vi "tare.vi"(0 "LC2 Tare\nAmount":dbl, 1 "Tare Pitot Tube\nNote: ONLY USE AT\nIDLE":bool, 2 "SYSTEM TARE\nONLY USE AT IDLE":bool, 3 "Tare LC1":bool, 4 "Previous \nAdjustment":dbl, 5 "Tare LC0":bool, 6 "LC0 Prev":dbl, 8 "AS 0":dbl, 9 "LC2 Prev":dbl, 10 "LC1 Tare \nAmount":dbl, 11 "LC1 Prev":dbl, 12 "LC0 Tare\nAmount":dbl, 13 "Tare LC2":bool, 14 "AS 1":dbl) -> (16 "AS0 Out":dbl, 18 "V_DIFF\nIndicator":dbl, 20 "LC1 Out":dbl, 21 "LC0 Out":dbl, 22 "Adjustment To Shift":dbl, 23 "LC2 Out":dbl, 24 "LC0 To\nShift":dbl, 25 "LC2 To \nShift":dbl, 26 "LC1 to \nShift":dbl)   [LabVIEW 2025]
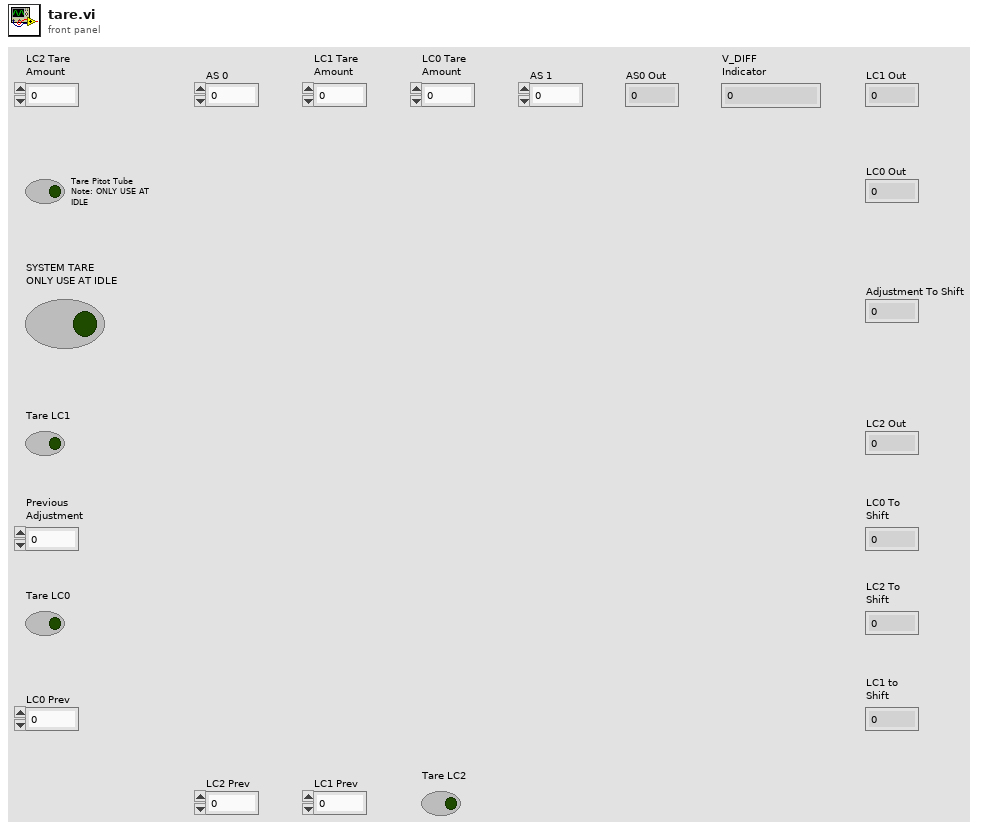
[diagram p1: front panel]
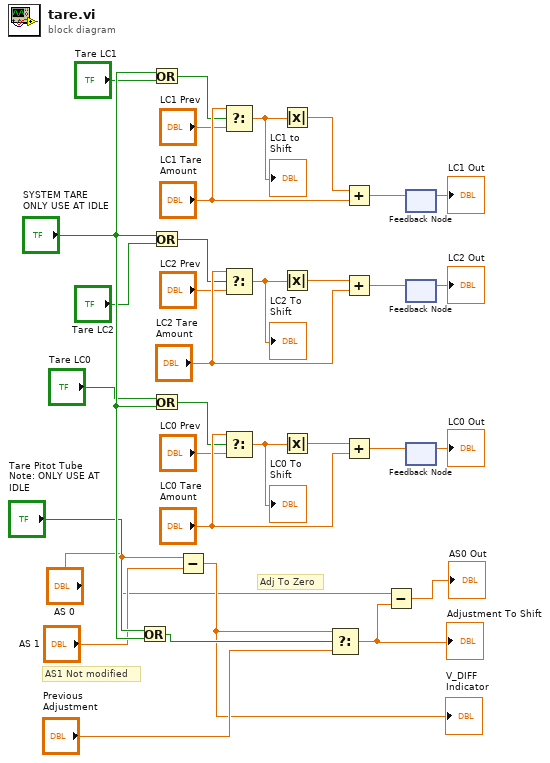
[diagram p0: block diagram]
diagram:
  # "AS1 Not modified"
  # "Adj To Zero"
  n1 = Or(x="Tare Pitot Tube\nNote: ONLY USE AT\nIDLE", y="SYSTEM TARE\nONLY USE AT IDLE") -> (x .or. y?=w20:bool)
  n2 = Or(x="SYSTEM TARE\nONLY USE AT IDLE", y="Tare LC1") -> (x .or. y?=w18:bool)
  n3 = Or(x="SYSTEM TARE\nONLY USE AT IDLE", y="Tare LC2") -> (x .or. y?=w19:bool)
  n4 = Or(x="Tare LC0", y="SYSTEM TARE\nONLY USE AT IDLE") -> (x .or. y?=w15:bool)
  n5 = Subtract(x="AS 0", y="AS 1") -> (x-y=w4:dbl)
  "V_DIFF\nIndicator" <- w4
  n6 = Select(t="LC1 Tare \nAmount", s=w18, f="LC1 Prev") -> (s? t:f=w27:dbl)
  "LC1 to \nShift" <- w27
  n7 = Select(t="LC2 Tare\nAmount", s=w19, f="LC2 Prev") -> (s? t:f=w29:dbl)
  "LC2 To \nShift" <- w29
  n8 = Select(t="LC0 Tare\nAmount", s=w15, f="LC0 Prev") -> (s? t:f=w25:dbl)
  "LC0 To\nShift" <- w25
  n9 = Absolute Value(x=w27) -> (abs(x)=w23:dbl)
  n10 = Absolute Value(x=w29) -> (abs(x)=w24:dbl)
  n11 = Absolute Value(x=w25) -> (abs(x)=w22:dbl)
  n12 = Select(t=w4, s=w20, f="Previous \nAdjustment") -> (s? t:f=w6:dbl)
  "Adjustment To Shift" <- w6
  n13 = Add(x=w23, y="LC1 Tare \nAmount") -> (x+y=w10:dbl)
  n14 = Add(x=w24, y="LC2 Tare\nAmount") -> (x+y=w9:dbl)
  n15 = Add(x=w22, y="LC0 Tare\nAmount") -> (x+y=w11:dbl)
  n16 = Subtract(x="AS 0", y=w6) -> (x-y=→"AS0 Out":dbl)
  n17 = feedback #1() -> (→"LC1 Out":dbl)  [unwired: 1 in]
  n18 = feedback-in #1(w10) -> ()
  n19 = feedback #2() -> (→"LC2 Out":dbl)  [unwired: 1 in]
  n20 = feedback-in #2(w9) -> ()
  n21 = feedback #3() -> (→"LC0 Out":dbl)  [unwired: 1 in]
  n22 = feedback-in #3(w11) -> ()
